vi "Destroy.vi"(8 "error in (no error)":errorcluster, 11 "test handler in":refnum<class "Test Handler.lvclass">) -> (0 "error out":errorcluster)   [LabVIEW 2018, in "Test Handler.lvclass"]
uses:
  Test Handler.lvclass
  Test Handler.lvclass/Test Handler.ctl
  src/api/extension/formatting_handler_interface/Formatting Handler.lvclass
panel:
  # "Connector Pane"
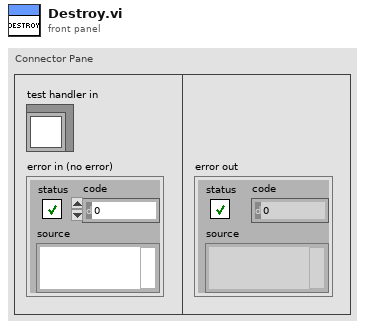
[diagram p1: front panel]
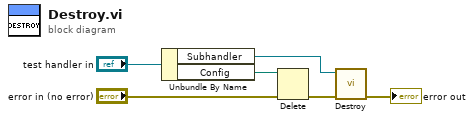
[diagram p0: block diagram]
diagram:
  n1 = Unbundle By Name("test handler in") -> ("Subhandler"=w3:refnum<class "Formatting Handler.lvclass">, "Config"=w5:path)
  n2 = Delete(path (use dialog)=w5, error in="error in (no error)") -> (error out=w2:errorcluster)  [unwired: 3 in, 2 out]
  n3 = call-dynamic "Destroy.vi"("error in (no error)"=w2, "handler in"=w3) -> ("error out"=→"error out":errorcluster)  [unwired: 9 in]
